vi "GetNodeMenuOptions.vi"(0 "reference":refnum<class "AbstractNode.lvclass">, 1 "MousePos":T1 {"y" format="%.2f"; "x" format="%.2f"}, 5 "error in (no error)":errorcluster) -> (14 "reference out":refnum<class "AbstractNode.lvclass">, 15 "MenuOptions":string[](array[string]), 19 "error out":errorcluster)   [LabVIEW 2020, in "AbstractNode.lvclass"]
uses:
  <resource>/Framework/Providers/Open_GDS/UML/AbstractNode_class/AbstractNode.lvclass
  <resource>/Framework/Providers/Open_GDS/UML/General/Point/Point Point2D.ctl
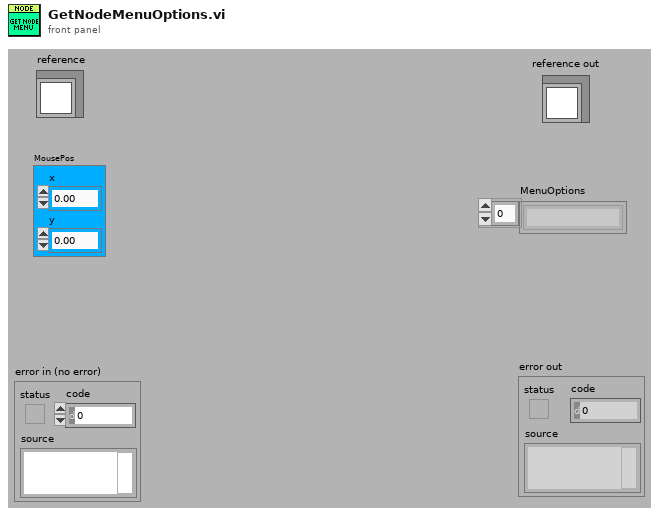
[diagram p1: front panel]
types:
  T1 = typedef "Point Point2D.ctl" = cluster{"x":dbl, "y":dbl}
  T2 = typedef "AbstractNode.lvclass/ObjectAttributes.ctl" = cluster{"parent":refnum<class "AbstractNode.lvclass">, "children":refnum<class "AbstractNode.lvclass">[], "Hidden":bool}
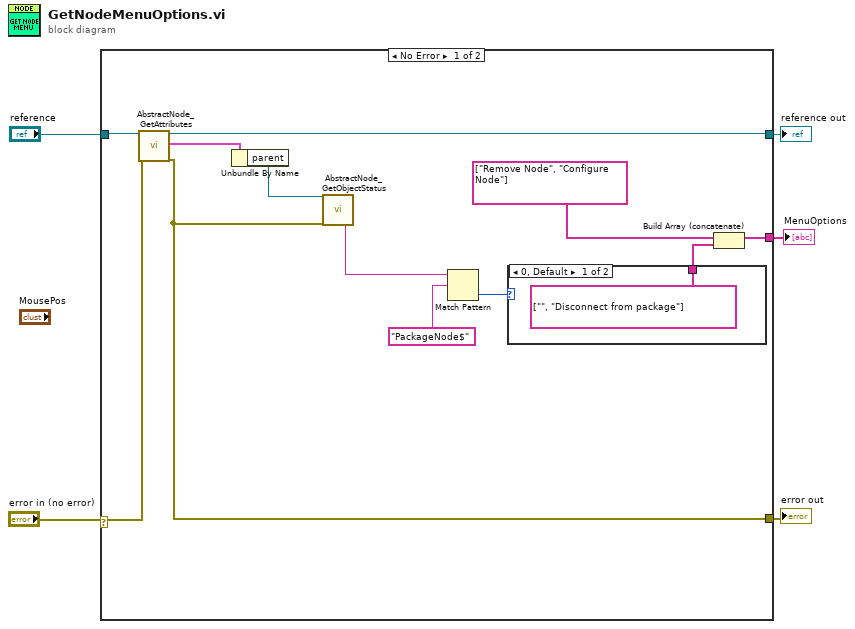
[diagram p0: block diagram]
diagram:
  n1 = case shown="No Error" "error in (no error)" {
    selector: "error in (no error)" -> [w16 w19]
    tunnel: "reference" -> [w17 w20]
    tunnel: [w11 w19] -> w4
    tunnel: [w14 w20] -> w3
    tunnel: [w8 _] -> w1
    frame No Error {
      n2 = call <resource>:"AbstractNode_GetAttributes.vi"("reference in"=w17, "error in (no error)"=w16) -> ("reference out"=w14:refnum<class "AbstractNode.lvclass">, "Data"=w7:T2, "error out"=w11:errorcluster)  [unwired: 14 in, 1 out]
      n3 = Unbundle By Name(w7) -> ("parent"=w13:refnum<class "AbstractNode.lvclass">)
      n4 = call <resource>:"AbstractNode_GetObjectStatus.vi"("reference in"=w13, "error in (no error)"=w11) -> ("Class name"=w6:string)  [unwired: 10 in, 7 out]
      n5 = Match Pattern(string=w6, regular expression="PackageNode$" ("y")) -> (offset past match=w12:i32)  [unwired: 4 out]
      n6 = case shown="0, Default" w12 {
        tunnel: [string[] ["", "Disconnect from package"] _] -> w9
        frame 0, Default {
        }
        frame -1 {
        }
      }
      n7 = Build Array (concatenate)(string[] ["Remove Node", "Configure Node"], w9) -> (w8:string[])
    }
    frame Error {
    }
  }
  "reference out" <- w3
  "error out" <- w4
  "MenuOptions" <- w1
